vi "Teach_Barcode.vi"() -> (0 "Teach Point:":T1 caption="教导点：", 1 "YESOrNO":bool)   [LabVIEW 2014]
uses:
  GTS/AxisControler.ctl
  <vilib>/Motion/FlexMotion/CustomControls/CustomControls.llb/AxisOrVectorSpaceControl To Control.flx
  axxon_Gold.vi
  <vilib>/vision/driver/NI_Vision_Acquisition_Software.lvlib
panel:
  in  "Radius":dbl caption="半径" min=0.0 max=10.0 step=0.1
  in  "Lighting Adjust":dbl(slide) caption="光源调节：" min=0.0 max=255.0 step=1.0 scale=0.0..255.0
  in  "Point":T1
  in  "TeachPoint":cluster{"X":dbl, "Y":dbl, "Z":dbl}
  out "Teach_Poition":cluster{"X":dbl, "Y":dbl}
  out "Image":T2(plugin-control)
  in  "CurrentTeachingPosition":T3
  in  "OK":bool
  in  "Concel":bool
  in  "JogPanel":T4
  in  "Heigh Speed:":dbl=20.0 caption="高速设定：" min=0.1 max=500.0 step=0.1 format="%#_4g"
  in  "Low Speed:":dbl=1.0 caption="低速设定：" min=0.1 max=500.0 step=0.1 format="%#_4g"
  # "(mm/s)"
  # "(mm/s)"
  # "Z"
  # "R"
  # "T"
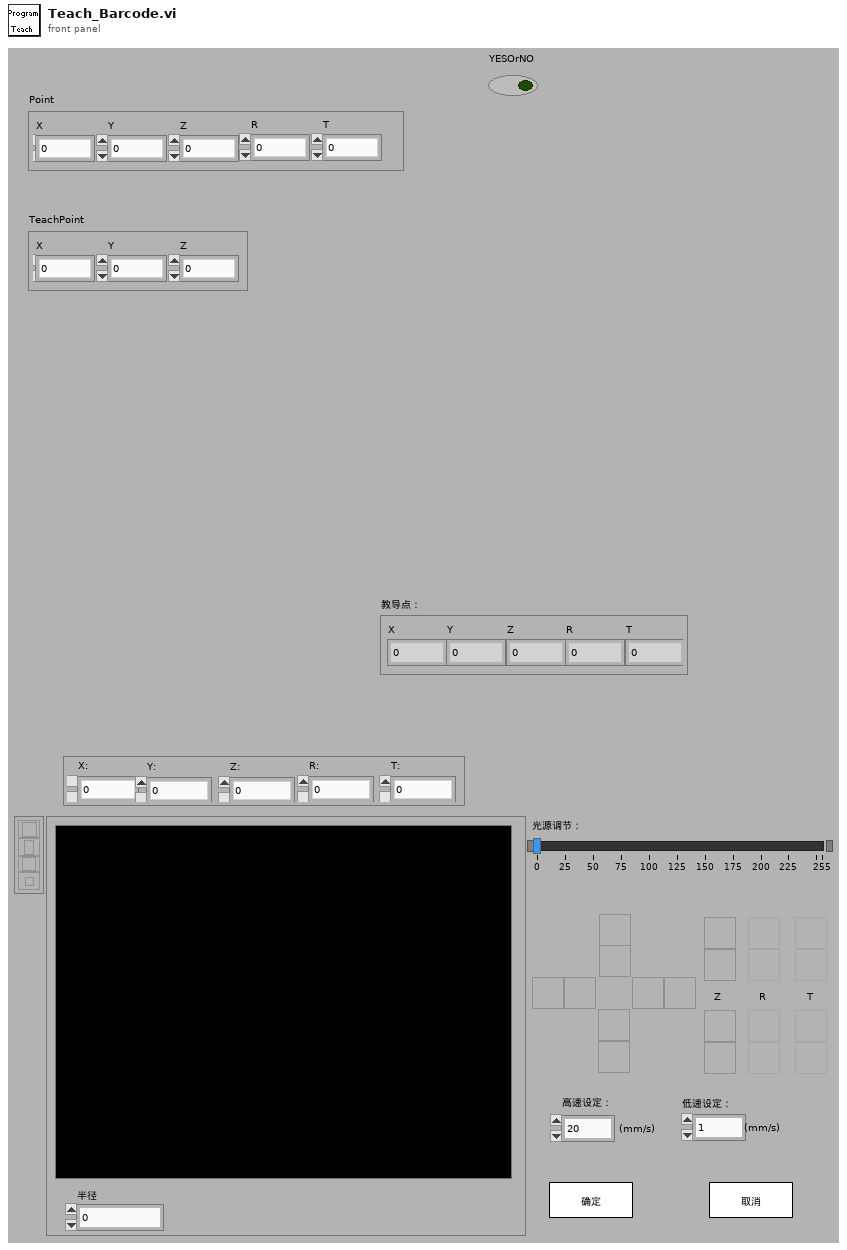
[diagram p1: front panel]
types:
  T1 = cluster{"X":dbl, "Y":dbl, "Z":dbl, "R":dbl, "T":dbl}
  T2 = typedef "IMAQ Image.ctl" = refnum<image>
  T3 = cluster{"X:":dbl, "Y:":dbl, "Z:":dbl, "R:":dbl, "T:":dbl}
  T4 = typedef "AxisControler.ctl" = cluster{"YFL":bool, "YFF":bool, "YBF":bool, "YBL":bool, "ZDF":bool, "ZDL":bool, "ZUL":bool, "ZUF":bool, "XRL":bool, "XRF":bool, "XLF":bool, "XLL":bool, "RPF":bool, "RPL":bool, "RNL":bool, "RNF":bool, "TPF":bool, "TPL":bool, "TNL":bool, "TNF":bool}
  T5 = enum8{"Enabled", "Disabled", "Disabled and Grayed Out"}
  T6 = cluster{"VISA resource name out":refnum<visa-resource-name>, "error out":errorcluster}
  T7 = cluster{"X Pulse Ratio":dbl, "Y Pulse Ratio":dbl, "Z Pulse Ratio":dbl, "X Lead":dbl, "Y Lead":dbl, "Z Lead":dbl, "Lead of adjusting motor":dbl, "Pulse Ratio of adjusting width motor":dbl, "Pulse Ratio of transfer motor":dbl, "Lead of transfer motor":dbl, "Solf limit of X axis":dbl, "Rotating Pulse Ratio":dbl, "Tilting Pulse Ratio":dbl, "Zeroing Position of Rotating axis":dbl, "Zeroing Position of Tilting axis":dbl, "LimitOfYAxis":dbl}
  T8 = typedef "IMAQdx.ctl" = refnum<k21>
  T9 = typedef "AxisOrVectorSpaceControl To Control.flx" = u16
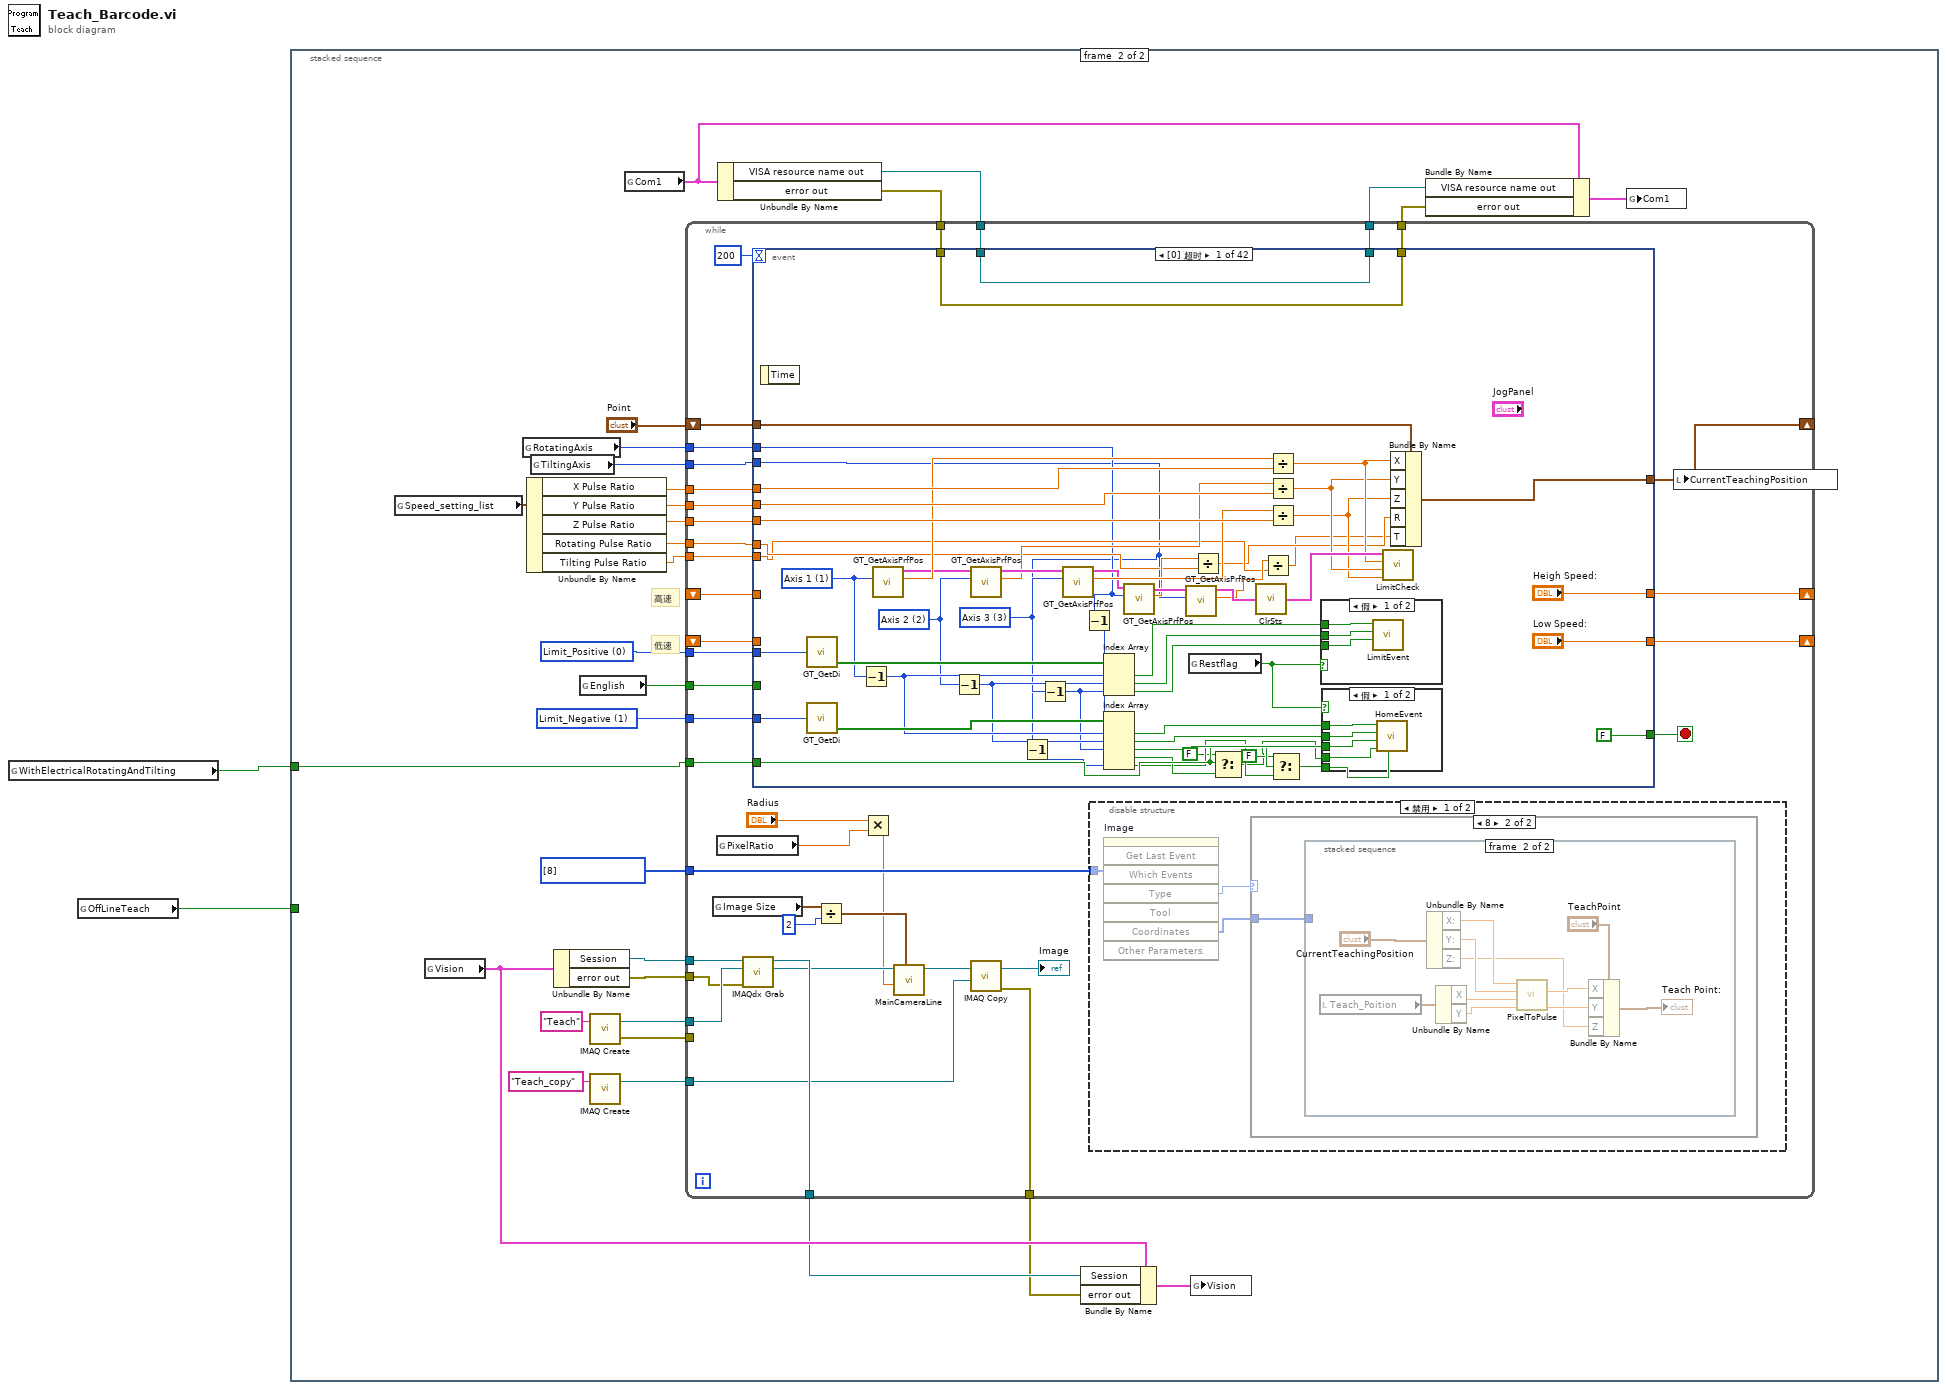
[diagram p0: block diagram]
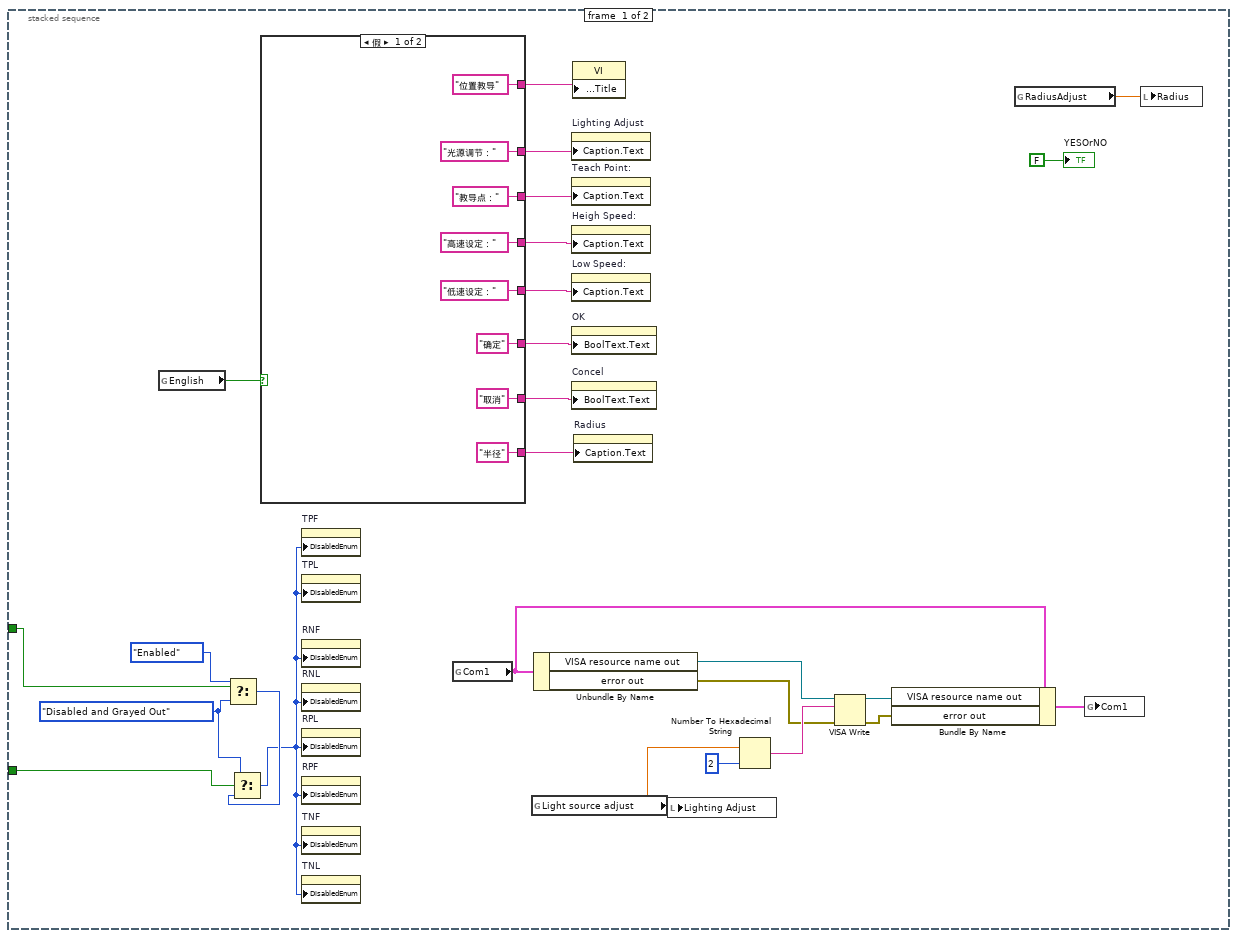
[diagram p2: hidden frame]
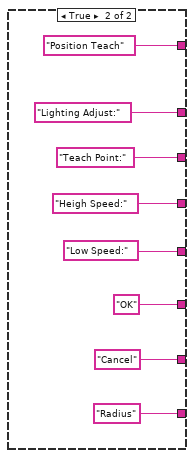
[diagram p3: hidden frame]
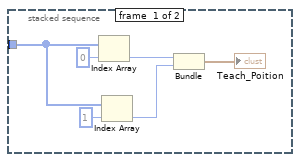
[diagram p5: hidden frame]
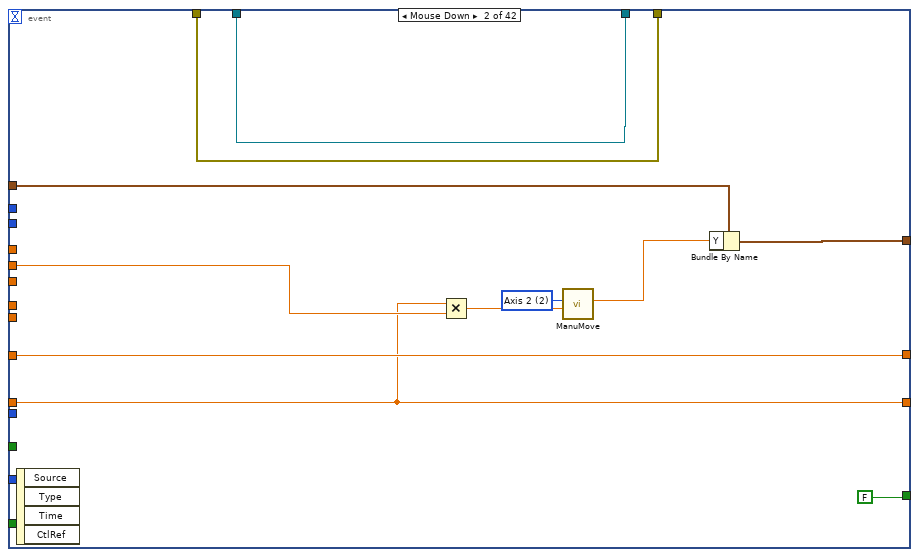
[diagram p9: hidden frame]
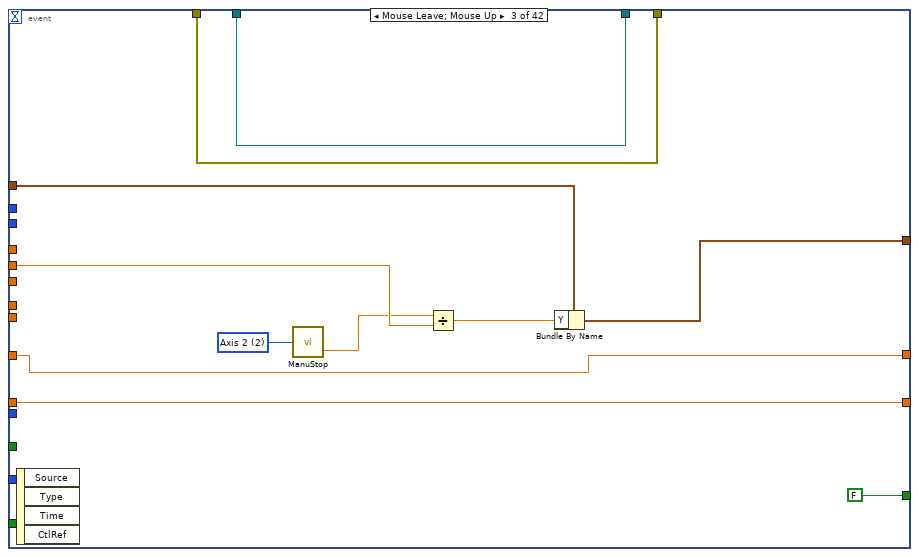
[diagram p10: hidden frame]
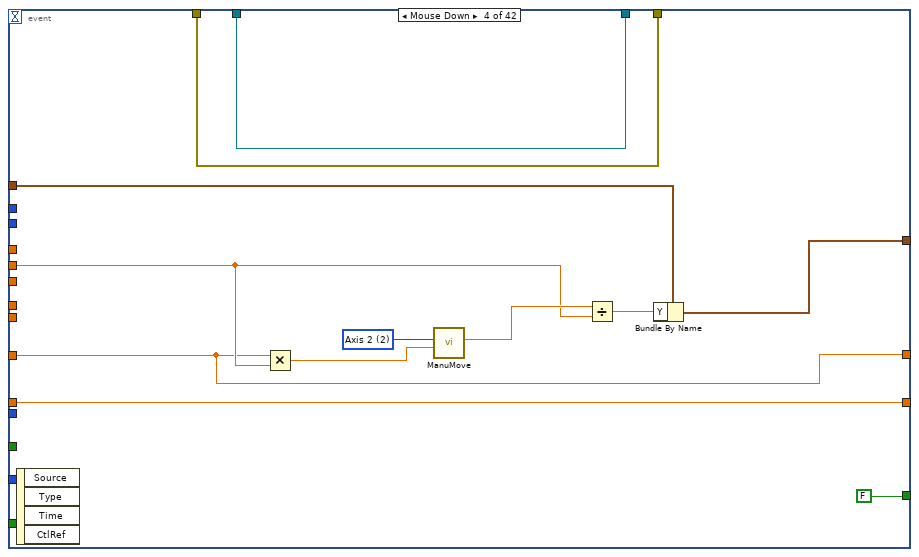
[diagram p11: hidden frame]
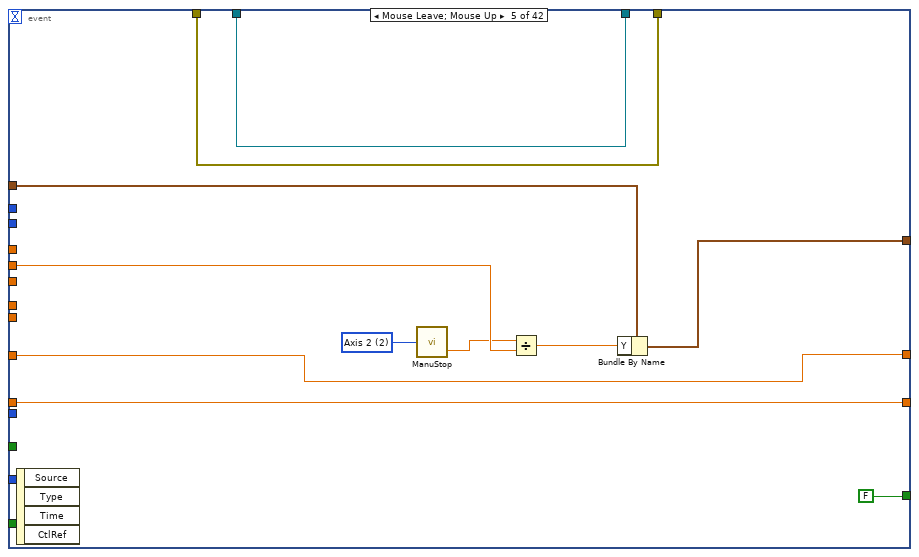
[diagram p12: hidden frame]
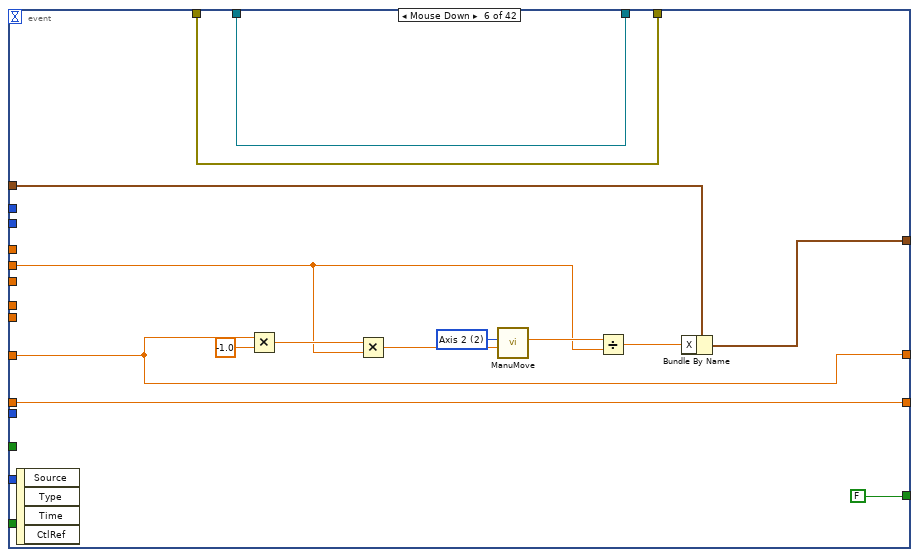
[diagram p13: hidden frame]
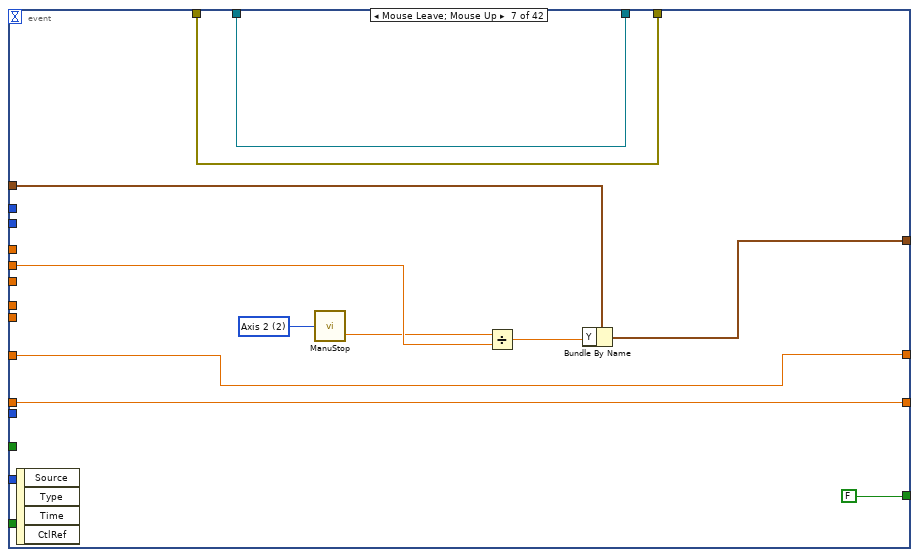
[diagram p14: hidden frame]
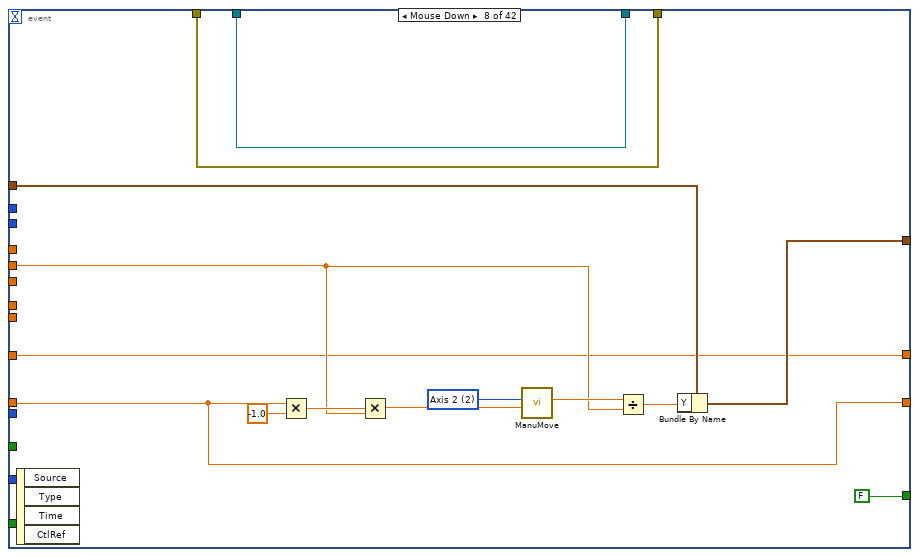
[diagram p15: hidden frame]
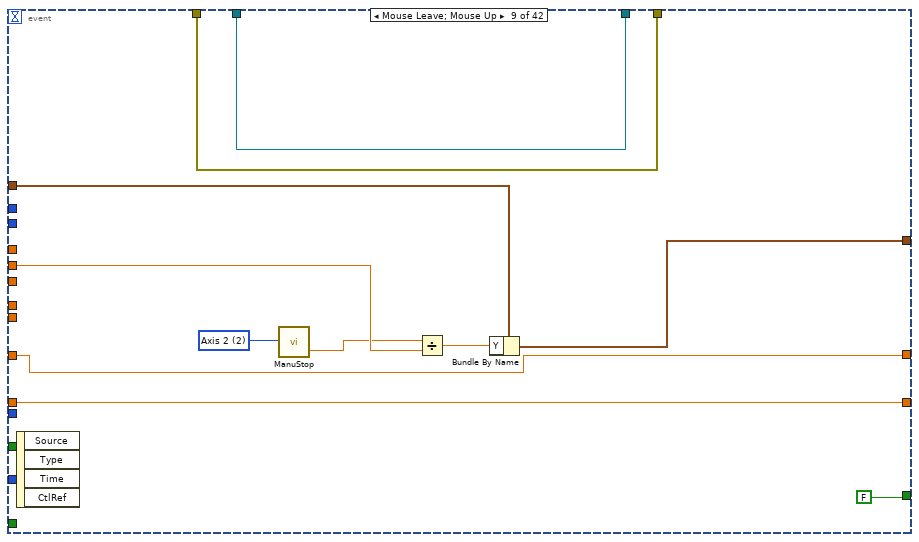
[diagram p16: hidden frame]
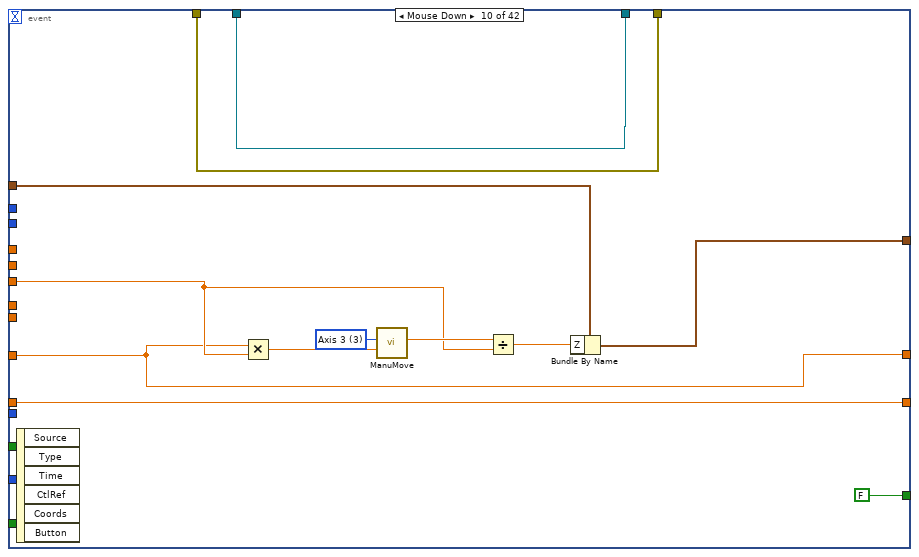
[diagram p17: hidden frame]
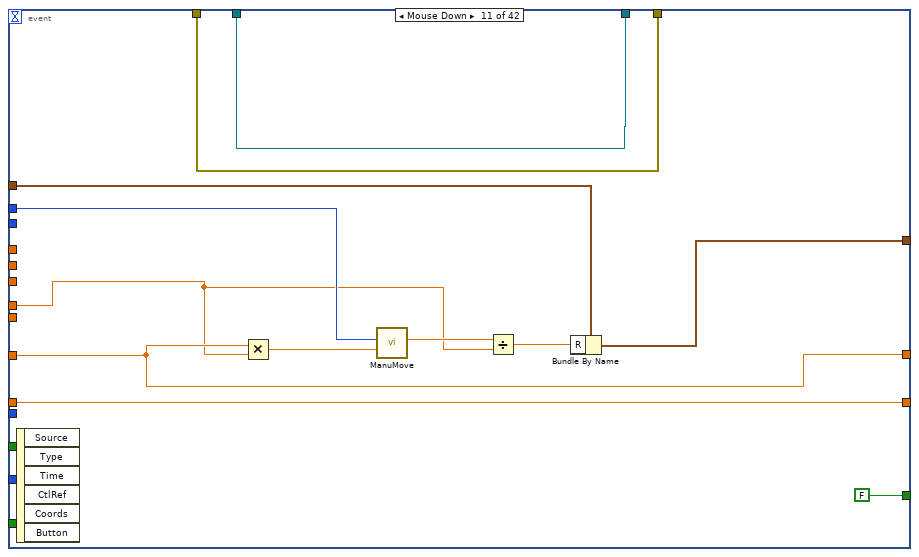
[diagram p18: hidden frame]
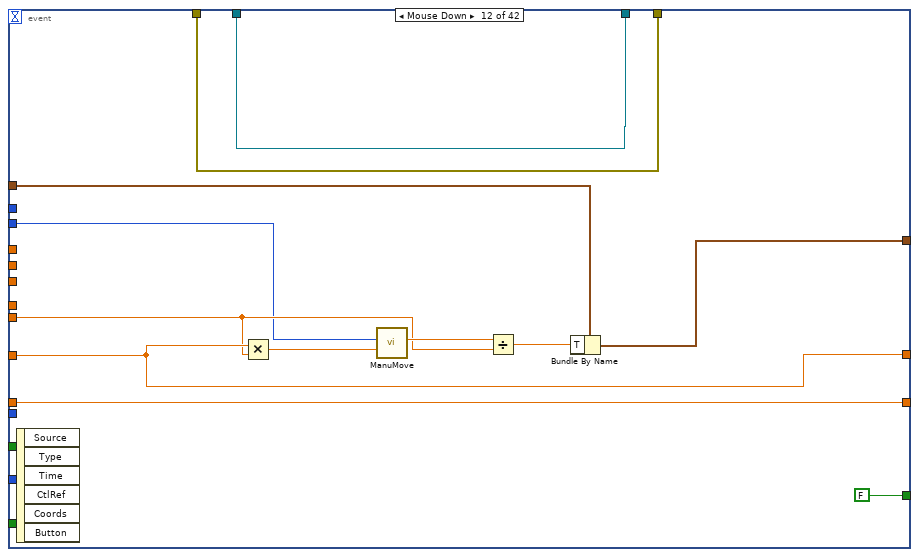
[diagram p19: hidden frame]
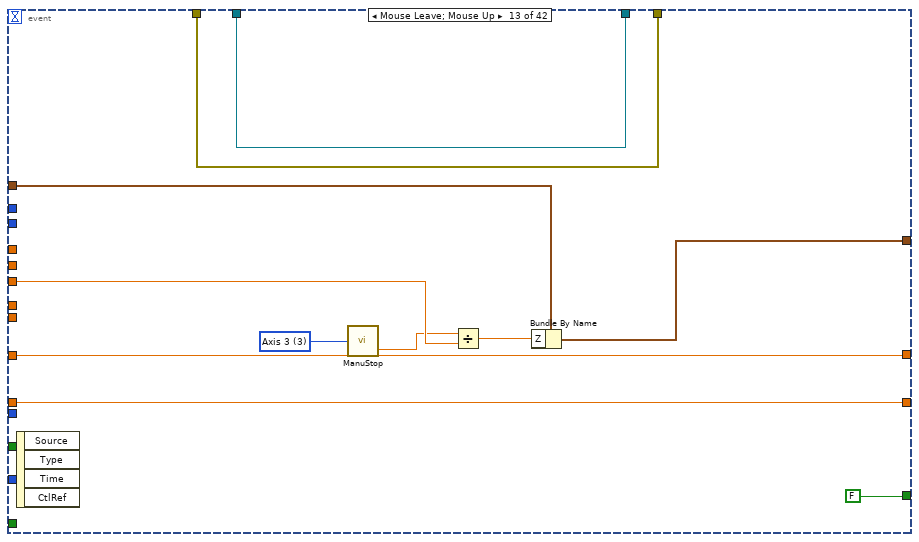
[diagram p20: hidden frame]
diagram:
  n1 = global read "axxon_Gold.vi" "WithElectricalRotatingAndTilting"() -> (w2:bool)
  n2 = global read "axxon_Gold.vi" "OffLineTeach"() -> (w1:bool)
  n3 = stacked-sequence {
    tunnel: w2 -> [w8 w46]
    tunnel: w1 -> [w6 _]
    frame #0 {
      w5 = T5."Disabled and Grayed Out" ("禁用")
      n4 = global read "axxon_Gold.vi" "English"() -> (w28:bool)
      n5 = Select(t=T5."Enabled" ("禁用"), s=w8, f=w5) -> (s? t:f=w4:T5)
      n6 = Select(t=w5, s=w6, f=w4) -> (s? t:f=w3:T5)
      n7 = case shown="假" w28 {
        tunnel: ["位置教导" ("前面板窗口:标题") "Position Teach" ("前面板窗口:标题")] -> w27
        tunnel: ["光源调节：" ("前面板窗口:标题") "Lighting Adjust:" ("前面板窗口:标题")] -> w26
        tunnel: ["教导点：" ("前面板窗口:标题") "Teach Point:" ("前面板窗口:标题")] -> w25
        tunnel: ["高速设定：" ("前面板窗口:标题") "Heigh Speed:" ("前面板窗口:标题")] -> w24
        tunnel: ["低速设定：" ("前面板窗口:标题") "Low Speed:" ("前面板窗口:标题")] -> w23
        tunnel: ["确定" ("前面板窗口:标题") "OK" ("前面板窗口:标题")] -> w22
        tunnel: ["取消" ("前面板窗口:标题") "Cancel" ("前面板窗口:标题")] -> w21
        tunnel: ["半径" ("前面板窗口:标题") "Radius" ("前面板窗口:标题")] -> w18
        frame False {
        }
        frame True {
        }
      }
      n8 = property on="TPF" class="Bool"("DisabledEnum"=w3) -> ()  [unwired: 2 in, 2 out]
      n9 = property on="TPL" class="Bool"("DisabledEnum"=w3) -> ()  [unwired: 2 in, 2 out]
      n10 = property on="RNF" class="Bool"("DisabledEnum"=w3) -> ()  [unwired: 2 in, 2 out]
      n11 = property on="RNL" class="Bool"("DisabledEnum"=w3) -> ()  [unwired: 2 in, 2 out]
      n12 = property on="RPL" class="Bool"("DisabledEnum"=w3) -> ()  [unwired: 2 in, 2 out]
      n13 = property on="RPF" class="Bool"("DisabledEnum"=w3) -> ()  [unwired: 2 in, 2 out]
      n14 = property on="TNF" class="Bool"("DisabledEnum"=w3) -> ()  [unwired: 2 in, 2 out]
      n15 = property on="TNL" class="Bool"("DisabledEnum"=w3) -> ()  [unwired: 2 in, 2 out]
      n16 = global read "axxon_Gold.vi" "Com1"() -> (w13:T6)
      n17 = global read "axxon_Gold.vi" "Light source adjust"() -> (w9:dbl)
      n18 = Unbundle By Name(w13) -> ("VISA resource name out"=w15:refnum<visa-resource-name>, "error out"=w14:errorcluster)
      n19 = property on="Lighting Adjust" class="Slide (严格)"("Caption.Text"=w26) -> ()  [unwired: 2 in, 2 out]
      n20 = property on="Teach Point:" class="Clust (严格)"("Caption.Text"=w25) -> ()  [unwired: 2 in, 2 out]
      n21 = property on="Heigh Speed:" class="DigNum (严格)"("Caption.Text"=w24) -> ()  [unwired: 2 in, 2 out]
      n22 = property on="Low Speed:" class="DigNum (严格)"("Caption.Text"=w23) -> ()  [unwired: 2 in, 2 out]
      n23 = property on="OK" class="Bool"("BoolText.Text"=w22) -> ()  [unwired: 2 in, 2 out]
      n24 = property on="Concel" class="Bool"("BoolText.Text"=w21) -> ()  [unwired: 2 in, 2 out]
      n25 = property class="VI"("Front Panel.Title"=w27) -> ()  [unwired: 2 in, 2 out]
      n26 = property on="Radius" class="DigNum (严格)"("Caption.Text"=w18) -> ()  [unwired: 2 in, 2 out]
      n27 = local write "Lighting Adjust"(w9) -> ()
      n28 = Number To Hexadecimal String(1:i16 2 ("宽度(-)"), 2:w9) -> (0:w17:string)
      n29 = VISA Write(VISA resource name=w15, write buffer=w17, error in (no error)=w14) -> (VISA resource name out=w12:refnum<visa-resource-name>, error out=w11:errorcluster)  [unwired: 1 out]
      n30 = Bundle By Name(cluster=w13, "VISA resource name out"=w12, "error out"=w11) -> (w10:T6)
      n31 = global read "axxon_Gold.vi" "RadiusAdjust"() -> (w19:dbl)
      n32 = global write "axxon_Gold.vi" "Com1"(w10) -> ()
      n33 = local write "Radius"(w19) -> ()
      "YESOrNO" <- FALSE ("确定YES?NO")
    }
    frame #1 {
      w51 = i16 1 items=["Limit_Positive", "Limit_Negative", "Alarm", "Home", "Gpi", "arrive"] ("diType in")
      w52 = i16 0 items=["Limit_Positive", "Limit_Negative", "Alarm", "Home", "Gpi", "arrive"] ("diType in")
      w69 = i32[] [8] items=["No  event", "Click event", "Draw event", "Move event", "Size event", "Scroll event", "Activate event", "Close event", "Double click event"] ("Events list (all)")
      # "低速"
      # "高速"
      n34 = global read "axxon_Gold.vi" "Speed_setting_list"() -> (w75:T7)
      n35 = global read "axxon_Gold.vi" "Vision"() -> (w64:cluster{"Session":T8, "error out":errorcluster})
      n36 = global read "axxon_Gold.vi" "RotatingAxis"() -> (w48:T9)
      n37 = Unbundle By Name(w75) -> ("X Pulse Ratio"=w74:dbl, "Y Pulse Ratio"=w73:dbl, "Z Pulse Ratio"=w72:dbl, "Rotating Pulse Ratio"=w50:dbl, "Tilting Pulse Ratio"=w49:dbl)
      n38 = global read "axxon_Gold.vi" "TiltingAxis"() -> (w47:T9)
      n39 = Unbundle By Name(w64) -> ("Session"=w66:T8, "error out"=w65:errorcluster)
      n40 = global read "axxon_Gold.vi" "English"() -> (w45:bool)
      n41 = call "IMAQ Create"("Image Name"="Teach") -> ("New Image"=w71:T2, "error out"=w70:errorcluster)  [unwired: 4 in]
      n42 = call "IMAQ Create"("Image Name"="Teach_copy") -> ("New Image"=w60:T2)  [unwired: 4 in, 1 out]
      n43 = global read "axxon_Gold.vi" "Com1"() -> (w53:T6)
      n44 = Unbundle By Name(w53) -> ("VISA resource name out"=w58:refnum<visa-resource-name>, "error out"=w57:errorcluster)
      n45 = while {
        tunnel: w74 -> [w114]
        tunnel: w73 -> [w113]
        tunnel: w72 -> [w112]
        tunnel: w71 -> [w110]
        tunnel: w70 -> [_]
        tunnel: w69 -> [w109]
        shift-right: [w108] -> _
        shift-left: _ -> [w104]
        shift-right: [w107] -> _
        shift-left: _ -> [w105]
        shift-right: [w102] -> _
        shift-left: "Point" -> [w106]
        tunnel: w58 -> [w101]
        tunnel: w57 -> [w100]
        tunnel: [w99] -> w56
        tunnel: [w98] -> w55
        tunnel: w66 -> [w97]
        tunnel: w65 -> [w96]
        tunnel: [w95] -> w63
        tunnel: w60 -> [w93]
        tunnel: [w92] -> w59
        tunnel: w52 -> [w89]
        tunnel: w51 -> [w88]
        tunnel: w50 -> [w86]
        tunnel: w49 -> [w87]
        tunnel: w48 -> [w85]
        tunnel: w47 -> [w84]
        tunnel: w46 -> [w83]
        tunnel: w45 -> [w82]
        stop <- w111 stop-if-true
        n46 = global read "axxon_Gold.vi" "Image Size"() -> (w81:cluster{"x":i32, "y":i32})
        n47 = global read "axxon_Gold.vi" "PixelRatio"() -> (w91:dbl)
        n48 = call <vilib>:"IMAQdx Grab.vi"("error in"=w96, "Image In"=w110, "Session In"=w97) -> ("Image Out"=w79:T2, "Session Out"=w95:T8)  [unwired: 5 in, 2 out]
        n49 = event shown="[0] 超时" {
          selector: _ -> [_ _ _ _ _ _ _ _ _ _ _ _ _ _ _ _ _ _ _ _ _ _ _ _ _ _ _ _ _ _ _ _ _ _ _ _ _ _ _ _ _ _]
          dyn-events: _ -> [_ _ _ _ _ _ _ _ _ _ _ _ _ _ _ _ _ _ _ _ _ _ _ _ _ _ _ _ _ _ _ _ _ _ _ _ _ _ _ _ _ _]
          timeout: 200 -> [_ _ _ _ _ _ _ _ _ _ _ _ _ _ _ _ _ _ _ _ _ _ _ _ _ _ _ _ _ _ _ _ _ _ _ _ _ _ _ _ _ _]
          tunnel: [FALSE FALSE FALSE FALSE FALSE FALSE FALSE FALSE FALSE FALSE FALSE FALSE FALSE FALSE FALSE FALSE FALSE FALSE FALSE FALSE FALSE FALSE FALSE FALSE FALSE FALSE FALSE FALSE FALSE FALSE FALSE FALSE FALSE FALSE FALSE TRUE FALSE FALSE TRUE TRUE w700 FALSE] -> w111
          tunnel: [w184 w207 w218 w231 w241 w252 w265 w277 w291 w302 w315 w327 w338 w351 w362 w371 w384 w396 w407 w418 w433 w447 w460 w471 w486 w500 w513 w524 w536 w547 w559 w570 w584 w595 w609 w621 w639 w659 w684 w698 w705 w728] -> w102
          tunnel: ["Heigh Speed:" w204 w215 w226 w238 w249 w263 w274 w288 w299 w312 w324 w335 w348 w359 w368 w381 w393 w404 w415 w430 w444 w457 w468 w483 w497 w510 w521 w533 w544 w556 w567 w581 w592 w606 w618 w636 w656 w681 w697 w702 w727] -> w108
          tunnel: ["Low Speed:" w203 w214 w225 w237 w248 w262 w273 w287 w298 w311 w323 w334 w347 w358 w367 w380 w392 w403 w414 w429 w443 w456 w467 w482 w496 w509 w520 w532 w543 w555 w566 w580 w591 w605 w617 w635 w655 w680 w696 w701 w726] -> w107
          tunnel: w114 -> [w188 _ _ _ _ _ _ _ _ _ _ _ _ _ _ _ _ _ _ _ _ _ _ _ _ _ _ w526 w538 w549 w561 w572 w586 w597 w611 _ _ _ _ _ _ _]
          tunnel: w113 -> [w187 w209 w220 w229 w243 w254 w267 w279 w293 _ _ _ _ _ _ _ _ _ _ _ _ _ _ _ _ _ _ _ _ _ _ _ _ _ _ _ _ _ _ _ _ _]
          tunnel: w112 -> [w186 _ _ _ _ _ _ _ _ w304 _ _ w340 _ _ w373 _ _ w409 w420 _ _ w462 w473 _ _ w515 _ _ _ _ _ _ _ _ _ _ _ _ _ _ _]
          tunnel: w106 -> [w185 w205 w216 w227 w239 w250 w264 w275 w289 w300 w313 w325 w336 w349 w360 w369 w382 w394 w405 w416 w431 w445 w458 w469 w484 w498 w511 w522 w534 w545 w557 w568 w582 w593 w607 w622 w640 w660 w685 w698 w706 w728]
          tunnel: w105 -> [_ w203 w214 w225 w237 w248 w262 w273 w287 w298 w311 w323 w334 w347 w358 w367 w380 w392 w403 w414 w429 w443 w456 w467 w482 w496 w509 w520 w532 w543 w555 w566 w580 w591 w605 w619 w637 w657 w682 w696 w703 w726]
          tunnel: w104 -> [_ w204 w215 w226 w238 w249 w263 w274 w288 w299 w312 w324 w335 w348 w359 w368 w381 w393 w404 w415 w430 w444 w457 w468 w483 w497 w510 w521 w533 w544 w556 w567 w581 w592 w606 w620 w638 w658 w683 w697 w704 w727]
          tunnel: w101 -> [w183 w202 w213 w224 w236 w247 w261 w272 w286 w297 w310 w322 w333 w346 w357 w366 w379 w391 w402 w413 w428 w442 w455 w466 w481 w495 w508 w519 w531 w542 w554 w565 w579 w590 w604 w616 w634 w654 w678 w694 w709 w723]
          tunnel: w100 -> [w182 w201 w212 w223 w235 w246 w260 w271 w285 w296 w309 w321 w332 w345 w356 w365 w378 w390 w401 w412 w427 w441 w454 w465 w480 w494 w507 w518 w530 w541 w553 w564 w578 w589 w603 w613 w631 w651 w676 w693 w707 w724]
          tunnel: [w183 w202 w213 w224 w236 w247 w261 w272 w286 w297 w310 w322 w333 w346 w357 w366 w379 w391 w402 w413 w428 w442 w455 w466 w481 w495 w508 w519 w531 w542 w554 w565 w579 w590 w604 w615 w633 w653 w679 w694 w710 w720] -> w99
          tunnel: [w182 w201 w212 w223 w235 w246 w260 w271 w285 w296 w309 w321 w332 w345 w356 w365 w378 w390 w401 w412 w427 w441 w454 w465 w480 w494 w507 w518 w530 w541 w553 w564 w578 w589 w603 w614 w632 w652 w677 w693 w708 w719] -> w98
          tunnel: w89 -> [w164 _ _ _ _ _ _ _ _ _ _ _ _ _ _ _ _ _ _ _ _ _ _ _ _ _ _ _ _ _ _ _ _ _ _ _ _ _ _ _ _ _]
          tunnel: w88 -> [w163 _ _ _ _ _ _ _ _ _ _ _ _ _ _ _ _ _ _ _ _ _ _ _ _ _ _ _ _ _ _ _ _ _ _ _ _ _ _ _ _ _]
          tunnel: w87 -> [w149 _ _ _ _ _ _ _ _ _ _ w320 _ _ w353 _ _ w389 _ _ _ w440 _ _ _ w493 _ _ _ _ _ _ _ _ _ _ _ _ _ _ _ _]
          tunnel: w86 -> [w150 _ _ _ _ _ _ _ _ _ w307 _ _ w342 _ _ w377 _ _ _ w426 _ _ _ w479 _ _ _ _ _ _ _ _ _ _ _ _ _ _ _ _ _]
          tunnel: w85 -> [w139 _ _ _ _ _ _ _ _ _ w308 _ _ w343 _ _ w376 _ _ _ w425 _ _ _ w478 _ _ _ _ _ _ _ _ _ _ _ _ _ _ _ _ _]
          tunnel: w84 -> [w138 _ _ _ _ _ _ _ _ _ _ w319 _ _ w354 _ _ w388 _ _ _ w439 _ _ _ w492 _ _ _ _ _ _ _ _ _ _ _ _ _ _ _ _]
          tunnel: w83 -> [w146 _ _ _ _ _ _ _ _ _ _ _ _ _ _ _ _ _ _ _ _ _ _ _ _ _ _ _ _ _ _ _ _ _ _ _ _ _ _ _ _ _]
          tunnel: w82 -> [_ _ _ _ _ _ _ _ _ _ _ _ _ _ _ _ _ _ _ _ _ _ _ _ _ _ _ _ _ _ _ _ _ _ _ _ _ w649 _ _ _ _]
          event Timeout {
            w169 = T9 3 items=["Axis Control"=0, "Axis 1"=1, "Axis 2"=2, "Axis 3"=3, "Axis 4"=4, "Axis 5"=5, "Axis 6"=6, "Axis 7"=7, "Axis 8"=8, "Vector Space Control"=16, "Vector Space 1"=17, "Vector Space 2"=18, "Vector Space 3"=19, "Vector Space 4"=20] ("Axis in")
            w171 = T9 2 items=["Axis Control"=0, "Axis 1"=1, "Axis 2"=2, "Axis 3"=3, "Axis 4"=4, "Axis 5"=5, "Axis 6"=6, "Axis 7"=7, "Axis 8"=8, "Vector Space Control"=16, "Vector Space 1"=17, "Vector Space 2"=18, "Vector Space 3"=19, "Vector Space 4"=20] ("Axis in")
            w173 = T9 1 items=["Axis Control"=0, "Axis 1"=1, "Axis 2"=2, "Axis 3"=3, "Axis 4"=4, "Axis 5"=5, "Axis 6"=6, "Axis 7"=7, "Axis 8"=8, "Vector Space Control"=16, "Vector Space 1"=17, "Vector Space 2"=18, "Vector Space 3"=19, "Vector Space 4"=20] ("Axis in")
            n50 = event-data() -> ()  [unwired: 1 in, 1 out]
            n51 = call "GT_GetDi.vi"("diType in"=w164) -> ("IOOut"=w175:bool[])  [unwired: 2 in, 2 out]
            n52 = call "GT_GetDi.vi"("diType in"=w163) -> ("IOOut"=w174:bool[])  [unwired: 2 in, 2 out]
            n53 = Decrement(x=w173) -> (x-1=w172:T9)
            n54 = call "GT_GetAxisPrfPos.vi"("Axis in"=w173) -> ("pValue"=w181:dbl, "rtn_Out"=w180:cluster{"rtn":i16, "Func":string})  [unwired: 6 in, 3 out]
            n55 = Decrement(x=w171) -> (x-1=w170:T9)
            n56 = call "GT_GetAxisPrfPos.vi"("Axis in"=w171, "rtn_In"=w180) -> ("pValue"=w178:dbl, "rtn_Out"=w179:cluster{"rtn":i16, "Func":string})  [unwired: 5 in, 3 out]
            n57 = Decrement(x=w138) -> (x-1=w136:T9)
            n58 = Decrement(x=w169) -> (x-1=w168:T9)
            n59 = call "GT_GetAxisPrfPos.vi"("Axis in"=w169, "rtn_In"=w179) -> ("pValue"=w177:dbl, "rtn_Out"=w154:cluster{"rtn":i16, "Func":string})  [unwired: 5 in, 3 out]
            n60 = Decrement(x=w139) -> (x-1=w137:T9)
            n61 = Index Array(array=w175, index #1=w172, index #2=w170, index #3=w168) -> (element #1=w167:bool, element #2=w166:bool, element #3=w165:bool)
            n62 = Index Array(array=w174, index #1=w172, index #2=w170, index #3=w168, index #4=w137, index #5=w136) -> (element #1=w162:bool, element #2=w161:bool, element #3=w160:bool, element #4=w145:bool, element #5=w144:bool)
            n63 = call "GT_GetAxisPrfPos.vi"("Axis in"=w139, "rtn_In"=w154) -> ("pValue"=w152:dbl, "rtn_Out"=w155:cluster{"rtn":i16, "Func":string})  [unwired: 5 in, 3 out]
            n64 = call "GT_GetAxisPrfPos.vi"("Axis in"=w138, "rtn_In"=w155) -> ("pValue"=w151:dbl, "rtn_Out"=w153:cluster{"rtn":i16, "Func":string})  [unwired: 5 in, 3 out]
            n65 = global read "axxon_Gold.vi" "Restflag"() -> (w176:bool)
            n66 = Divide(x=w152, y=w150) -> (x/y=w148:dbl)
            n67 = Select(t=FALSE, s=w146, f=w145) -> (s? t:f=w141:bool)
            n68 = call "ClrSts.vi"("rtn_In"=w153) -> ("rtn_Out"=w159:cluster{"rtn":i16, "Func":string})
            n69 = Divide(x=w151, y=w149) -> (x/y=w147:dbl)
            n70 = Divide(x=w181, y=w188) -> (x/y=w158:dbl)
            n71 = Divide(x=w178, y=w187) -> (x/y=w157:dbl)
            n72 = Divide(x=w177, y=w186) -> (x/y=w156:dbl)
            n73 = Select(t=FALSE, s=w146, f=w144) -> (s? t:f=w140:bool)
            n74 = case shown="假" w176 {
              tunnel: w167 -> [w199 _]
              tunnel: w166 -> [w198 _]
              tunnel: w165 -> [w197 _]
              frame False {
                n75 = call "LimitEvent.vi"("Z Limit"=w197, "Y Limit"=w198, "X Limit"=w199) -> ()  [unwired: 8 in]
              }
              frame True {
              }
            }
            n76 = case shown="假" w176 {
              tunnel: w162 -> [w196 _]
              tunnel: w161 -> [w195 _]
              tunnel: w160 -> [w194 _]
              tunnel: w141 -> [w193 _]
              tunnel: w140 -> [w192 _]
              frame False {
                n77 = call "HomeEvent.vi"("T Home"=w192, "R Home"=w193, "Z Home"=w194, "Y Home"=w195, "X Home"=w196) -> ()  [unwired: 6 in]
              }
              frame True {
              }
            }
            n78 = call "LimitCheck.vi"("Z"=w156, "Y"=w157, "X"=w158, "rtn_In"=w159) -> ()  [unwired: 3 in, 1 out]
            n79 = Bundle By Name(cluster=w185, "X"=w158, "Y"=w157, "Z"=w156, "R"=w148, "T"=w147) -> (w184:T1)
          }
          event Mouse Down {
            w200 = T9 2 items=["Axis Control"=0, "Axis 1"=1, "Axis 2"=2, "Axis 3"=3, "Axis 4"=4, "Axis 5"=5, "Axis 6"=6, "Axis 7"=7, "Axis 8"=8, "Vector Space Control"=16, "Vector Space 1"=17, "Vector Space 2"=18, "Vector Space 3"=19, "Vector Space 4"=20] ("Axis in")
            n80 = event-data() -> ()  [unwired: 1 in, 4 out]
            n81 = Multiply(x=w203, y=w209) -> (x*y=w210:dbl)
            n82 = call "ManuMove.vi"("Velocity"=w210, "Axis in"=w200) -> ("Position"=w208:dbl)  [unwired: 5 in, 1 out]
            n83 = Bundle By Name(cluster=w205, "Y"=w208) -> (w207:T1)
          }
          event Mouse Leave; Mouse Up {
            w221 = T9 2 items=["Axis Control"=0, "Axis 1"=1, "Axis 2"=2, "Axis 3"=3, "Axis 4"=4, "Axis 5"=5, "Axis 6"=6, "Axis 7"=7, "Axis 8"=8, "Vector Space Control"=16, "Vector Space 1"=17, "Vector Space 2"=18, "Vector Space 3"=19, "Vector Space 4"=20] ("Axis")
            n84 = event-data() -> ()  [unwired: 1 in, 4 out]
            n85 = call "ManuStop.vi"("Axis in"=w221) -> ("Position"=w211:dbl)  [unwired: 2 in, 1 out]
            n86 = Divide(x=w211, y=w220) -> (x/y=w219:dbl)
            n87 = Bundle By Name(cluster=w216, "Y"=w219) -> (w218:T1)
          }
          event Mouse Down {
            w222 = T9 2 items=["Axis Control"=0, "Axis 1"=1, "Axis 2"=2, "Axis 3"=3, "Axis 4"=4, "Axis 5"=5, "Axis 6"=6, "Axis 7"=7, "Axis 8"=8, "Vector Space Control"=16, "Vector Space 1"=17, "Vector Space 2"=18, "Vector Space 3"=19, "Vector Space 4"=20] ("Axis in")
            n88 = event-data() -> ()  [unwired: 1 in, 4 out]
            n89 = Multiply(x=w226, y=w229) -> (x*y=w228:dbl)
            n90 = call "ManuMove.vi"("Velocity"=w228, "Axis in"=w222) -> ("Position"=w233:dbl)  [unwired: 5 in, 1 out]
            n91 = Divide(x=w233, y=w229) -> (x/y=w232:dbl)
            n92 = Bundle By Name(cluster=w227, "Y"=w232) -> (w231:T1)
          }
          event Mouse Leave; Mouse Up {
            w244 = T9 2 items=["Axis Control"=0, "Axis 1"=1, "Axis 2"=2, "Axis 3"=3, "Axis 4"=4, "Axis 5"=5, "Axis 6"=6, "Axis 7"=7, "Axis 8"=8, "Vector Space Control"=16, "Vector Space 1"=17, "Vector Space 2"=18, "Vector Space 3"=19, "Vector Space 4"=20] ("Axis")
            n93 = event-data() -> ()  [unwired: 1 in, 4 out]
            n94 = call "ManuStop.vi"("Axis in"=w244) -> ("Position"=w234:dbl)  [unwired: 2 in, 1 out]
            n95 = Divide(x=w234, y=w243) -> (x/y=w242:dbl)
            n96 = Bundle By Name(cluster=w239, "Y"=w242) -> (w241:T1)
          }
          event Mouse Down {
            w245 = T9 2 items=["Axis Control"=0, "Axis 1"=1, "Axis 2"=2, "Axis 3"=3, "Axis 4"=4, "Axis 5"=5, "Axis 6"=6, "Axis 7"=7, "Axis 8"=8, "Vector Space Control"=16, "Vector Space 1"=17, "Vector Space 2"=18, "Vector Space 3"=19, "Vector Space 4"=20] ("Axis in")
            n97 = event-data() -> ()  [unwired: 1 in, 4 out]
            n98 = Multiply(x=w249, y=-1.0) -> (x*y=w257:dbl)
            n99 = Multiply(x=w257, y=w254) -> (x*y=w258:dbl)
            n100 = call "ManuMove.vi"("Velocity"=w258, "Axis in"=w245) -> ("Position"=w255:dbl)  [unwired: 5 in, 1 out]
            n101 = Divide(x=w255, y=w254) -> (x/y=w253:dbl)
            n102 = Bundle By Name(cluster=w250, "X"=w253) -> (w252:T1)
          }
          event Mouse Leave; Mouse Up {
            w268 = T9 2 items=["Axis Control"=0, "Axis 1"=1, "Axis 2"=2, "Axis 3"=3, "Axis 4"=4, "Axis 5"=5, "Axis 6"=6, "Axis 7"=7, "Axis 8"=8, "Vector Space Control"=16, "Vector Space 1"=17, "Vector Space 2"=18, "Vector Space 3"=19, "Vector Space 4"=20] ("Axis")
            n103 = event-data() -> ()  [unwired: 1 in, 4 out]
            n104 = call "ManuStop.vi"("Axis in"=w268) -> ("Position"=w259:dbl)  [unwired: 2 in, 1 out]
            n105 = Divide(x=w259, y=w267) -> (x/y=w266:dbl)
            n106 = Bundle By Name(cluster=w264, "Y"=w266) -> (w265:T1)
          }
          event Mouse Down {
            w270 = T9 2 items=["Axis Control"=0, "Axis 1"=1, "Axis 2"=2, "Axis 3"=3, "Axis 4"=4, "Axis 5"=5, "Axis 6"=6, "Axis 7"=7, "Axis 8"=8, "Vector Space Control"=16, "Vector Space 1"=17, "Vector Space 2"=18, "Vector Space 3"=19, "Vector Space 4"=20] ("Axis in")
            n107 = event-data() -> ()  [unwired: 1 in, 4 out]
            n108 = Multiply(x=w273, y=-1.0) -> (x*y=w282:dbl)
            n109 = Multiply(x=w282, y=w279) -> (x*y=w283:dbl)
            n110 = call "ManuMove.vi"("Velocity"=w283, "Axis in"=w270) -> ("Position"=w280:dbl)  [unwired: 5 in, 1 out]
            n111 = Divide(x=w280, y=w279) -> (x/y=w278:dbl)
            n112 = Bundle By Name(cluster=w275, "Y"=w278) -> (w277:T1)
          }
          event Mouse Leave; Mouse Up {
            w294 = T9 2 items=["Axis Control"=0, "Axis 1"=1, "Axis 2"=2, "Axis 3"=3, "Axis 4"=4, "Axis 5"=5, "Axis 6"=6, "Axis 7"=7, "Axis 8"=8, "Vector Space Control"=16, "Vector Space 1"=17, "Vector Space 2"=18, "Vector Space 3"=19, "Vector Space 4"=20] ("Axis")
            n113 = event-data() -> ()  [unwired: 1 in, 4 out]
            n114 = call "ManuStop.vi"("Axis in"=w294) -> ("Position"=w284:dbl)  [unwired: 2 in, 1 out]
            n115 = Divide(x=w284, y=w293) -> (x/y=w292:dbl)
            n116 = Bundle By Name(cluster=w289, "Y"=w292) -> (w291:T1)
          }
          event Mouse Down {
            w295 = T9 3 items=["Axis Control"=0, "Axis 1"=1, "Axis 2"=2, "Axis 3"=3, "Axis 4"=4, "Axis 5"=5, "Axis 6"=6, "Axis 7"=7, "Axis 8"=8, "Vector Space Control"=16, "Vector Space 1"=17, "Vector Space 2"=18, "Vector Space 3"=19, "Vector Space 4"=20] ("Axis in")
            n117 = event-data() -> ()  [unwired: 1 in, 6 out]
            n118 = Multiply(x=w299, y=w304) -> (x*y=w306:dbl)
            n119 = call "ManuMove.vi"("Velocity"=w306, "Axis in"=w295) -> ("Position"=w305:dbl)  [unwired: 5 in, 1 out]
            n120 = Divide(x=w305, y=w304) -> (x/y=w303:dbl)
            n121 = Bundle By Name(cluster=w300, "Z"=w303) -> (w302:T1)
          }
          event Mouse Down {
            n122 = event-data() -> ()  [unwired: 1 in, 6 out]
            n123 = Multiply(x=w312, y=w307) -> (x*y=w318:dbl)
            n124 = call "ManuMove.vi"("Velocity"=w318, "Axis in"=w308) -> ("Position"=w317:dbl)  [unwired: 5 in, 1 out]
            n125 = Divide(x=w317, y=w307) -> (x/y=w316:dbl)
            n126 = Bundle By Name(cluster=w313, "R"=w316) -> (w315:T1)
          }
          event Mouse Down {
            n127 = event-data() -> ()  [unwired: 1 in, 6 out]
            n128 = Multiply(x=w324, y=w320) -> (x*y=w330:dbl)
            n129 = call "ManuMove.vi"("Velocity"=w330, "Axis in"=w319) -> ("Position"=w329:dbl)  [unwired: 5 in, 1 out]
            n130 = Divide(x=w329, y=w320) -> (x/y=w328:dbl)
            n131 = Bundle By Name(cluster=w325, "T"=w328) -> (w327:T1)
          }
          event Mouse Leave; Mouse Up {
            w341 = T9 3 items=["Axis Control"=0, "Axis 1"=1, "Axis 2"=2, "Axis 3"=3, "Axis 4"=4, "Axis 5"=5, "Axis 6"=6, "Axis 7"=7, "Axis 8"=8, "Vector Space Control"=16, "Vector Space 1"=17, "Vector Space 2"=18, "Vector Space 3"=19, "Vector Space 4"=20] ("Axis")
            n132 = event-data() -> ()  [unwired: 1 in, 4 out]
            n133 = call "ManuStop.vi"("Axis in"=w341) -> ("Position"=w331:dbl)  [unwired: 2 in, 1 out]
            n134 = Divide(x=w331, y=w340) -> (x/y=w339:dbl)
            n135 = Bundle By Name(cluster=w336, "Z"=w339) -> (w338:T1)
          }
          event Mouse Leave; Mouse Up {
            n136 = event-data() -> ()  [unwired: 1 in, 4 out]
            n137 = call "ManuStop.vi"("Axis in"=w343) -> ("Position"=w344:dbl)  [unwired: 2 in, 1 out]
            n138 = Divide(x=w344, y=w342) -> (x/y=w352:dbl)
            n139 = Bundle By Name(cluster=w349, "R"=w352) -> (w351:T1)
          }
          event Mouse Leave; Mouse Up {
            n140 = event-data() -> ()  [unwired: 1 in, 4 out]
            n141 = call "ManuStop.vi"("Axis in"=w354) -> ("Position"=w355:dbl)  [unwired: 2 in, 1 out]
            n142 = Divide(x=w355, y=w353) -> (x/y=w363:dbl)
            n143 = Bundle By Name(cluster=w360, "T"=w363) -> (w362:T1)
          }
          event Mouse Down {
            w364 = T9 3 items=["Axis Control"=0, "Axis 1"=1, "Axis 2"=2, "Axis 3"=3, "Axis 4"=4, "Axis 5"=5, "Axis 6"=6, "Axis 7"=7, "Axis 8"=8, "Vector Space Control"=16, "Vector Space 1"=17, "Vector Space 2"=18, "Vector Space 3"=19, "Vector Space 4"=20] ("Axis in")
            n144 = event-data() -> ()  [unwired: 1 in, 6 out]
            n145 = Multiply(x=w367, y=w373) -> (x*y=w375:dbl)
            n146 = call "ManuMove.vi"("Velocity"=w375, "Axis in"=w364) -> ("Position"=w374:dbl)  [unwired: 5 in, 1 out]
            n147 = Divide(x=w374, y=w373) -> (x/y=w372:dbl)
            n148 = Bundle By Name(cluster=w369, "Z"=w372) -> (w371:T1)
          }
          event Mouse Down {
            n149 = event-data() -> ()  [unwired: 1 in, 6 out]
            n150 = Multiply(x=w380, y=w377) -> (x*y=w387:dbl)
            n151 = call "ManuMove.vi"("Velocity"=w387, "Axis in"=w376) -> ("Position"=w386:dbl)  [unwired: 5 in, 1 out]
            n152 = Divide(x=w386, y=w377) -> (x/y=w385:dbl)
            n153 = Bundle By Name(cluster=w382, "R"=w385) -> (w384:T1)
          }
          event Mouse Down {
            n154 = event-data() -> ()  [unwired: 1 in, 6 out]
            n155 = Multiply(x=w392, y=w389) -> (x*y=w399:dbl)
            n156 = call "ManuMove.vi"("Velocity"=w399, "Axis in"=w388) -> ("Position"=w398:dbl)  [unwired: 5 in, 1 out]
            n157 = Divide(x=w398, y=w389) -> (x/y=w397:dbl)
            n158 = Bundle By Name(cluster=w394, "T"=w397) -> (w396:T1)
          }
          event Mouse Leave; Mouse Up {
            w410 = T9 3 items=["Axis Control"=0, "Axis 1"=1, "Axis 2"=2, "Axis 3"=3, "Axis 4"=4, "Axis 5"=5, "Axis 6"=6, "Axis 7"=7, "Axis 8"=8, "Vector Space Control"=16, "Vector Space 1"=17, "Vector Space 2"=18, "Vector Space 3"=19, "Vector Space 4"=20] ("Axis")
            n159 = event-data() -> ()  [unwired: 1 in, 4 out]
            n160 = call "ManuStop.vi"("Axis in"=w410) -> ("Position"=w400:dbl)  [unwired: 2 in, 1 out]
            n161 = Divide(x=w400, y=w409) -> (x/y=w408:dbl)
            n162 = Bundle By Name(cluster=w405, "Z"=w408) -> (w407:T1)
          }
          event Mouse Down {
            w411 = T9 3 items=["Axis Control"=0, "Axis 1"=1, "Axis 2"=2, "Axis 3"=3, "Axis 4"=4, "Axis 5"=5, "Axis 6"=6, "Axis 7"=7, "Axis 8"=8, "Vector Space Control"=16, "Vector Space 1"=17, "Vector Space 2"=18, "Vector Space 3"=19, "Vector Space 4"=20] ("Axis in")
            n163 = event-data() -> ()  [unwired: 1 in, 6 out]
            n164 = Multiply(x=w414, y=-1.0) -> (x*y=w423:dbl)
            n165 = Multiply(x=w423, y=w420) -> (x*y=w422:dbl)
            n166 = call "ManuMove.vi"("Velocity"=w422, "Axis in"=w411) -> ("Position"=w421:dbl)  [unwired: 5 in, 1 out]
            n167 = Divide(x=w421, y=w420) -> (x/y=w419:dbl)
            n168 = Bundle By Name(cluster=w416, "Z"=w419) -> (w418:T1)
          }
          event Mouse Down {
            n169 = event-data() -> ()  [unwired: 1 in, 6 out]
            n170 = Multiply(x=w429, y=-1.0) -> (x*y=w437:dbl)
            n171 = Multiply(x=w437, y=w426) -> (x*y=w436:dbl)
            n172 = call "ManuMove.vi"("Velocity"=w436, "Axis in"=w425) -> ("Position"=w435:dbl)  [unwired: 5 in, 1 out]
            n173 = Divide(x=w435, y=w426) -> (x/y=w434:dbl)
            n174 = Bundle By Name(cluster=w431, "R"=w434) -> (w433:T1)
          }
          event Mouse Down {
            n175 = event-data() -> ()  [unwired: 1 in, 6 out]
            n176 = Multiply(x=w443, y=-1.0) -> (x*y=w451:dbl)
            n177 = Multiply(x=w451, y=w440) -> (x*y=w450:dbl)
            n178 = call "ManuMove.vi"("Velocity"=w450, "Axis in"=w439) -> ("Position"=w449:dbl)  [unwired: 5 in, 1 out]
            n179 = Divide(x=w449, y=w440) -> (x/y=w448:dbl)
            n180 = Bundle By Name(cluster=w445, "T"=w448) -> (w447:T1)
          }
          event Mouse Leave; Mouse Up {
            w463 = T9 3 items=["Axis Control"=0, "Axis 1"=1, "Axis 2"=2, "Axis 3"=3, "Axis 4"=4, "Axis 5"=5, "Axis 6"=6, "Axis 7"=7, "Axis 8"=8, "Vector Space Control"=16, "Vector Space 1"=17, "Vector Space 2"=18, "Vector Space 3"=19, "Vector Space 4"=20] ("Axis")
            n181 = event-data() -> ()  [unwired: 1 in, 4 out]
            n182 = call "ManuStop.vi"("Axis in"=w463) -> ("Position"=w453:dbl)  [unwired: 2 in, 1 out]
            n183 = Divide(x=w453, y=w462) -> (x/y=w461:dbl)
            n184 = Bundle By Name(cluster=w458, "Z"=w461) -> (w460:T1)
          }
          event Mouse Down {
            w464 = T9 3 items=["Axis Control"=0, "Axis 1"=1, "Axis 2"=2, "Axis 3"=3, "Axis 4"=4, "Axis 5"=5, "Axis 6"=6, "Axis 7"=7, "Axis 8"=8, "Vector Space Control"=16, "Vector Space 1"=17, "Vector Space 2"=18, "Vector Space 3"=19, "Vector Space 4"=20] ("Axis in")
            n185 = event-data() -> ()  [unwired: 1 in, 6 out]
            n186 = Multiply(x=w468, y=-1.0) -> (x*y=w476:dbl)
            n187 = Multiply(x=w476, y=w473) -> (x*y=w475:dbl)
            n188 = call "ManuMove.vi"("Velocity"=w475, "Axis in"=w464) -> ("Position"=w474:dbl)  [unwired: 5 in, 1 out]
            n189 = Divide(x=w474, y=w473) -> (x/y=w472:dbl)
            n190 = Bundle By Name(cluster=w469, "Z"=w472) -> (w471:T1)
          }
          event Mouse Down {
            n191 = event-data() -> ()  [unwired: 1 in, 6 out]
            n192 = Multiply(x=w483, y=-1.0) -> (x*y=w490:dbl)
            n193 = Multiply(x=w490, y=w479) -> (x*y=w489:dbl)
            n194 = call "ManuMove.vi"("Velocity"=w489, "Axis in"=w478) -> ("Position"=w488:dbl)  [unwired: 5 in, 1 out]
            n195 = Divide(x=w488, y=w479) -> (x/y=w487:dbl)
            n196 = Bundle By Name(cluster=w484, "R"=w487) -> (w486:T1)
          }
          event Mouse Down {
            n197 = event-data() -> ()  [unwired: 1 in, 6 out]
            n198 = Multiply(x=w497, y=-1.0) -> (x*y=w504:dbl)
            n199 = Multiply(x=w504, y=w493) -> (x*y=w503:dbl)
            n200 = call "ManuMove.vi"("Velocity"=w503, "Axis in"=w492) -> ("Position"=w502:dbl)  [unwired: 5 in, 1 out]
            n201 = Divide(x=w502, y=w493) -> (x/y=w501:dbl)
            n202 = Bundle By Name(cluster=w498, "T"=w501) -> (w500:T1)
          }
          event Mouse Leave; Mouse Up {
            w516 = T9 3 items=["Axis Control"=0, "Axis 1"=1, "Axis 2"=2, "Axis 3"=3, "Axis 4"=4, "Axis 5"=5, "Axis 6"=6, "Axis 7"=7, "Axis 8"=8, "Vector Space Control"=16, "Vector Space 1"=17, "Vector Space 2"=18, "Vector Space 3"=19, "Vector Space 4"=20] ("Axis")
            n203 = event-data() -> ()  [unwired: 1 in, 4 out]
            n204 = call "ManuStop.vi"("Axis in"=w516) -> ("Position"=w506:dbl)  [unwired: 2 in, 1 out]
            n205 = Divide(x=w506, y=w515) -> (x/y=w514:dbl)
            n206 = Bundle By Name(cluster=w511, "Z"=w514) -> (w513:T1)
          }
          event Mouse Down {
            w517 = T9 1 items=["Axis Control"=0, "Axis 1"=1, "Axis 2"=2, "Axis 3"=3, "Axis 4"=4, "Axis 5"=5, "Axis 6"=6, "Axis 7"=7, "Axis 8"=8, "Vector Space Control"=16, "Vector Space 1"=17, "Vector Space 2"=18, "Vector Space 3"=19, "Vector Space 4"=20] ("Axis in")
            n207 = event-data() -> ()  [unwired: 1 in, 6 out]
            n208 = Multiply(x=w520, y=w526) -> (x*y=w528:dbl)
            n209 = call "ManuMove.vi"("Velocity"=w528, "Axis in"=w517) -> ("Position"=w527:dbl)  [unwired: 5 in, 1 out]
            n210 = Divide(x=w527, y=w526) -> (x/y=w525:dbl)
            n211 = Bundle By Name(cluster=w522, "X"=w525) -> (w524:T1)
          }
          event Mouse Leave; Mouse Up {
            w539 = T9 1 items=["Axis Control"=0, "Axis 1"=1, "Axis 2"=2, "Axis 3"=3, "Axis 4"=4, "Axis 5"=5, "Axis 6"=6, "Axis 7"=7, "Axis 8"=8, "Vector Space Control"=16, "Vector Space 1"=17, "Vector Space 2"=18, "Vector Space 3"=19, "Vector Space 4"=20] ("Axis")
            n212 = event-data() -> ()  [unwired: 1 in, 4 out]
            n213 = call "ManuStop.vi"("Axis in"=w539) -> ("Position"=w529:dbl)  [unwired: 2 in, 1 out]
            n214 = Divide(x=w529, y=w538) -> (x/y=w537:dbl)
            n215 = Bundle By Name(cluster=w534, "X"=w537) -> (w536:T1)
          }
          event Mouse Down {
            w540 = T9 1 items=["Axis Control"=0, "Axis 1"=1, "Axis 2"=2, "Axis 3"=3, "Axis 4"=4, "Axis 5"=5, "Axis 6"=6, "Axis 7"=7, "Axis 8"=8, "Vector Space Control"=16, "Vector Space 1"=17, "Vector Space 2"=18, "Vector Space 3"=19, "Vector Space 4"=20] ("Axis in")
            n216 = event-data() -> ()  [unwired: 1 in, 6 out]
            n217 = Multiply(x=w544, y=w549) -> (x*y=w550:dbl)
            n218 = call "ManuMove.vi"("Velocity"=w550, "Axis in"=w540) -> ("Position"=w551:dbl)  [unwired: 5 in, 1 out]
            n219 = Divide(x=w551, y=w549) -> (x/y=w548:dbl)
            n220 = Bundle By Name(cluster=w545, "X"=w548) -> (w547:T1)
          }
          event Mouse Leave; Mouse Up {
            w562 = T9 1 items=["Axis Control"=0, "Axis 1"=1, "Axis 2"=2, "Axis 3"=3, "Axis 4"=4, "Axis 5"=5, "Axis 6"=6, "Axis 7"=7, "Axis 8"=8, "Vector Space Control"=16, "Vector Space 1"=17, "Vector Space 2"=18, "Vector Space 3"=19, "Vector Space 4"=20] ("Axis")
            n221 = event-data() -> ()  [unwired: 1 in, 4 out]
            n222 = call "ManuStop.vi"("Axis in"=w562) -> ("Position"=w552:dbl)  [unwired: 2 in, 1 out]
            n223 = Divide(x=w552, y=w561) -> (x/y=w560:dbl)
            n224 = Bundle By Name(cluster=w557, "X"=w560) -> (w559:T1)
          }
          event Mouse Down {
            w563 = T9 1 items=["Axis Control"=0, "Axis 1"=1, "Axis 2"=2, "Axis 3"=3, "Axis 4"=4, "Axis 5"=5, "Axis 6"=6, "Axis 7"=7, "Axis 8"=8, "Vector Space Control"=16, "Vector Space 1"=17, "Vector Space 2"=18, "Vector Space 3"=19, "Vector Space 4"=20] ("Axis in")
            n225 = event-data() -> ()  [unwired: 1 in, 6 out]
            n226 = Multiply(x=w567, y=-1.0) -> (x*y=w575:dbl)
            n227 = Multiply(x=w575, y=w572) -> (x*y=w574:dbl)
            n228 = call "ManuMove.vi"("Velocity"=w574, "Axis in"=w563) -> ("Position"=w573:dbl)  [unwired: 5 in, 1 out]
            n229 = Divide(x=w573, y=w572) -> (x/y=w571:dbl)
            n230 = Bundle By Name(cluster=w568, "X"=w571) -> (w570:T1)
          }
          event Mouse Leave; Mouse Up {
            w587 = T9 1 items=["Axis Control"=0, "Axis 1"=1, "Axis 2"=2, "Axis 3"=3, "Axis 4"=4, "Axis 5"=5, "Axis 6"=6, "Axis 7"=7, "Axis 8"=8, "Vector Space Control"=16, "Vector Space 1"=17, "Vector Space 2"=18, "Vector Space 3"=19, "Vector Space 4"=20] ("Axis")
            n231 = event-data() -> ()  [unwired: 1 in, 4 out]
            n232 = call "ManuStop.vi"("Axis in"=w587) -> ("Position"=w577:dbl)  [unwired: 2 in, 1 out]
            n233 = Divide(x=w577, y=w586) -> (x/y=w585:dbl)
            n234 = Bundle By Name(cluster=w582, "X"=w585) -> (w584:T1)
          }
          event Mouse Down {
            w588 = T9 1 items=["Axis Control"=0, "Axis 1"=1, "Axis 2"=2, "Axis 3"=3, "Axis 4"=4, "Axis 5"=5, "Axis 6"=6, "Axis 7"=7, "Axis 8"=8, "Vector Space Control"=16, "Vector Space 1"=17, "Vector Space 2"=18, "Vector Space 3"=19, "Vector Space 4"=20] ("Axis in")
            n235 = event-data() -> ()  [unwired: 1 in, 7 out]
            n236 = Multiply(x=w591, y=-1.0) -> (x*y=w600:dbl)
            n237 = Multiply(x=w600, y=w597) -> (x*y=w599:dbl)
            n238 = call "ManuMove.vi"("Velocity"=w599, "Axis in"=w588) -> ("Position"=w598:dbl)  [unwired: 5 in, 1 out]
            n239 = Divide(x=w598, y=w597) -> (x/y=w596:dbl)
            n240 = Bundle By Name(cluster=w593, "X"=w596) -> (w595:T1)
          }
          event Mouse Leave; Mouse Up {
            w612 = T9 1 items=["Axis Control"=0, "Axis 1"=1, "Axis 2"=2, "Axis 3"=3, "Axis 4"=4, "Axis 5"=5, "Axis 6"=6, "Axis 7"=7, "Axis 8"=8, "Vector Space Control"=16, "Vector Space 1"=17, "Vector Space 2"=18, "Vector Space 3"=19, "Vector Space 4"=20] ("Axis")
            n241 = event-data() -> ()  [unwired: 1 in, 4 out]
            n242 = call "ManuStop.vi"("Axis in"=w612) -> ("Position"=w602:dbl)  [unwired: 2 in, 1 out]
            n243 = Divide(x=w602, y=w611) -> (x/y=w610:dbl)
            n244 = Bundle By Name(cluster=w607, "X"=w610) -> (w609:T1)
          }
          event "Concel": Value Change {
            n245 = event-data() -> ()  [unwired: 1 in, 6 out]
            n246 = stacked-sequence {
              tunnel: w622 -> [w629]
              tunnel: [w629] -> w621
              tunnel: w620 -> [w628]
              tunnel: w619 -> [w627]
              tunnel: [w628] -> w618
              tunnel: [w627] -> w617
              tunnel: w616 -> [w625]
              tunnel: [w625] -> w615
              tunnel: [w624] -> w614
              tunnel: w613 -> [w624]
              frame #0 {
                n247 = local write "YESOrNO"(FALSE ("确定YES?NO")) -> ()
              }
            }
          }
          event "Image": Shortcut Menu Selection (User) {
            n248 = event-data() -> ("ItemTag"=w630:string)  [unwired: 1 in, 7 out]
            n249 = stacked-sequence {
              tunnel: w640 -> [_ w648]
              tunnel: [_ w648] -> w639
              tunnel: w638 -> [_ w647]
              tunnel: w637 -> [_ w646]
              tunnel: [_ w647] -> w636
              tunnel: [_ w646] -> w635
              tunnel: w634 -> [_ w645]
              tunnel: [_ w645] -> w633
              tunnel: [_ w644] -> w632
              tunnel: w631 -> [_ w644]
              tunnel: w630 -> [w642 _]
              frame #0 {
                n250 = case shown="\"ZoomToFit\"" w642 {
                  frame "假", Default {
                  }
                  frame "ZoomToFit" {
                    n251 = property on="Image" class="ImageControl"("Zoom to Fit Mode"=TRUE) -> ()  [unwired: 2 in, 2 out]
                  }
                }
              }
              frame #1 {
              }
            }
          }
          event "Image": Shortcut Menu Activation? {
            n252 = event-data() -> ("MenuRef"=w650:refnum<k9>)  [unwired: 1 in, 4 out]
            n253 = stacked-sequence {
              tunnel: w660 -> [_ w675]
              tunnel: [_ w675] -> w659
              tunnel: w658 -> [_ w674]
              tunnel: w657 -> [_ w673]
              tunnel: [_ w674] -> w656
              tunnel: [_ w673] -> w655
              tunnel: w654 -> [_ w672]
              tunnel: [_ w672] -> w653
              tunnel: [_ w671] -> w652
              tunnel: w651 -> [_ w671]
              tunnel: w650 -> [w667 _]
              tunnel: w649 -> [w668 _]
              tunnel: [w662 _] -> _
              frame #0 {
                n254 = case shown="假" w668 {
                  tunnel: [string[] ["匹配大小"] ("项名称") string[] ["Zoom To Fit"] ("项名称")] -> w664
                  frame False {
                  }
                  frame True {
                  }
                }
                n255 = Delete Menu Items(9:w667) -> (0:w663:errorcluster, 3:w666:refnum<k9>)  [unwired: 3 in]
                n256 = Insert Menu Items(6:w663, 7:string[] ["ZoomToFit"] ("项标识符"), 8:w664, 9:w666) -> (0:w662:errorcluster)  [unwired: 2 in, 2 out]
              }
              frame #1 {
              }
            }
            n257 = event-data() -> ()  [unwired: 2 in, 1 out]
          }
          event "OK": Value Change {
            n258 = event-data() -> ()  [unwired: 1 in, 6 out]
            n259 = stacked-sequence {
              tunnel: w685 -> [w687 _]
              tunnel: [w687 _] -> w684
              tunnel: w683 -> [_ w692]
              tunnel: w682 -> [_ w691]
              tunnel: [_ w692] -> w681
              tunnel: [_ w691] -> w680
              tunnel: [_ w690] -> w679
              tunnel: w678 -> [_ w690]
              tunnel: [_ w689] -> w677
              tunnel: w676 -> [_ w689]
              frame #0 {
                n260 = local write "Teach Point:"(w687) -> ()
                n261 = local write "YESOrNO"(TRUE ("确定YES?NO")) -> ()
              }
              frame #1 {
              }
            }
          }
          event Panel Close {
            n262 = event-data() -> ()  [unwired: 1 in, 4 out]
            n263 = local write "YESOrNO"(FALSE ("确定YES?NO")) -> ()
          }
          event "Radius": Value Change {
            n264 = event-data() -> ()  [unwired: 1 in, 6 out]
            n265 = stacked-sequence {
              tunnel: [_ w717] -> w710
              tunnel: w709 -> [_ w717]
              tunnel: [_ w716] -> w708
              tunnel: w707 -> [_ w716]
              tunnel: w706 -> [_ w715]
              tunnel: [_ w715] -> w705
              tunnel: w704 -> [_ w714]
              tunnel: w703 -> [_ w713]
              tunnel: [_ w714] -> w702
              tunnel: [_ w713] -> w701
              tunnel: [_ FALSE] -> w700
              frame #0 {
              }
              frame #1 {
                n266 = local read "Radius"() -> (w711:dbl)
                n267 = global write "axxon_Gold.vi" "RadiusAdjust"(w711) -> ()
              }
            }
          }
          event "Lighting Adjust": Value Change {
            n268 = event-data() -> ()  [unwired: 1 in, 6 out]
            n269 = flat-sequence {
              tunnel: w724 -> [w735]
              tunnel: w723 -> [w736]
              tunnel: [w733] -> w722
              tunnel: [w732] -> w721
              tunnel: [w731] -> w718
              tunnel: w722 -> [w738]
              tunnel: w721 -> [w737]
              tunnel: [w738] -> w720
              tunnel: [w737] -> w719
              tunnel: w718 -> [_]
              frame #0 {
                n270 = global write "axxon_Gold.vi" "Light source adjust"("Lighting Adjust") -> ()
                n271 = Number To Hexadecimal String(1:i16 2 ("宽度(-)"), 2:"Lighting Adjust") -> (0:w734:string)
                n272 = VISA Write(VISA resource name=w736, write buffer=w734, error in (no error)=w735) -> (VISA resource name out=w733:refnum<visa-resource-name>, return count=w731:u32, error out=w732:errorcluster)
              }
              frame #1 {
                n273 = Wait (ms)(milliseconds to wait=u32 20 ("等待时间（毫秒）")) -> ()  [unwired: 1 out]
              }
            }
          }
        }
        n274 = Divide(x=w81, y=2) -> (x/y=w77:cluster{"x":dbl, "y":dbl})
        n275 = Multiply(x="Radius", y=w91) -> (x*y=w76:dbl)
        n276 = call "MainCameraLine.vi"("ImageCentral"=w77, "R"=w76, "Image"=w79) -> ("Image Out"=w78:T2)  [unwired: 7 in, 1 out]
        n277 = call "IMAQ Copy"("Image Dst"=w93, "Image Src"=w78) -> ("error out"=w92:errorcluster, "Image Dst Out"=→"Image":T2)  [unwired: 4 in]
        n278 = disable-structure shown="禁用" {
          disable-tunnel: w109 -> [w117 _]
          frame Disabled {
            n279 = invoke on="Image" class="ImageControl" method="Get Last Event"("Which Events"=w117) -> ("Type"=w116:i32, "Coordinates"=w115:i32[])  [unwired: 7 in, 6 out]
            n280 = case shown="8" w116 {
              tunnel: w115 -> [_ w118]
              frame 0, Default {
              }
              frame 8 {
                n281 = stacked-sequence {
                  tunnel: w118 -> [w123 _]
                  frame #0 {
                    n282 = Index Array(array=w123, index=0 ("索引")) -> (element=w121:i32)
                    n283 = Index Array(array=w123, index=1 ("索引")) -> (element=w120:i32)
                    n284 = Bundle(w121, w120) -> (→"Teach_Poition":cluster{i32, i32})  [unwired: 1 in]
                  }
                  frame #1 {
                    n285 = local read "Teach_Poition"() -> (w130:cluster{"X":dbl, "Y":dbl})
                    n286 = Unbundle By Name("CurrentTeachingPosition") -> ("X:"=w132:dbl, "Y:"=w131:dbl, "Z:"=w126:dbl)
                    n287 = Unbundle By Name(w130) -> ("X"=w135:dbl, "Y"=w134:dbl)
                    n288 = call "PixelToPulse.vi"("PixelY"=w134, "PixelX"=w135, "IN Y"=w131, "IN X"=w132) -> ("Out Y"=w127:dbl, "Out X"=w128:dbl)  [unwired: 1 in, 2 out]
                    n289 = Bundle By Name(cluster="TeachPoint", "X"=w128, "Y"=w127, "Z"=w126) -> (→"Teach Point:":cluster{"X":dbl, "Y":dbl, "Z":dbl})
                  }
                }
              }
            }
          }
          frame Enabled {
          }
        }
        n290 = local write "CurrentTeachingPosition"(w102) -> ()
      }
      n291 = Bundle By Name(cluster=w64, "Session"=w63, "error out"=w59) -> (w62:cluster{"Session":T8, "error out":errorcluster})
      n292 = global write "axxon_Gold.vi" "Vision"(w62) -> ()
      n293 = Bundle By Name(cluster=w53, "VISA resource name out"=w56, "error out"=w55) -> (w54:T6)
      n294 = global write "axxon_Gold.vi" "Com1"(w54) -> ()
    }
  }
